vi "Set Object Bounds.vi"(5 "Resize Only? [F]":bool, 7 "Position Only? [F]":bool, 8 "error in (no error)":errorcluster, 9 "rect":T1, 11 "GObject":refnum<vi>) -> (0 "error out":errorcluster, 3 "DUP GObject":refnum<vi>)   [LabVIEW 2013, in "IObject.lvclass"]
uses:
  IObject.lvclass
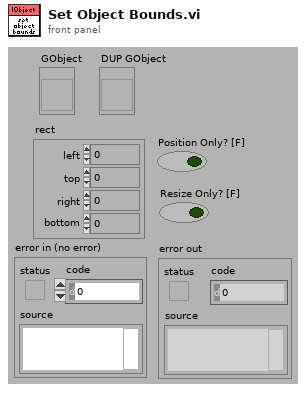
[diagram p1: front panel]
types:
  T1 = cluster{"left":dbl, "top":dbl, "right":dbl, "bottom":dbl}
  T2 = cluster{"left":bool, "top":bool, "right":bool, "bottom":bool}
  T3 = cluster{"left":i32, "top":i32, "right":i32, "bottom":i32}
  T4 = typedef "LVPositionTypeDef.ctl" = cluster{"Left":i32, "Top":i32}
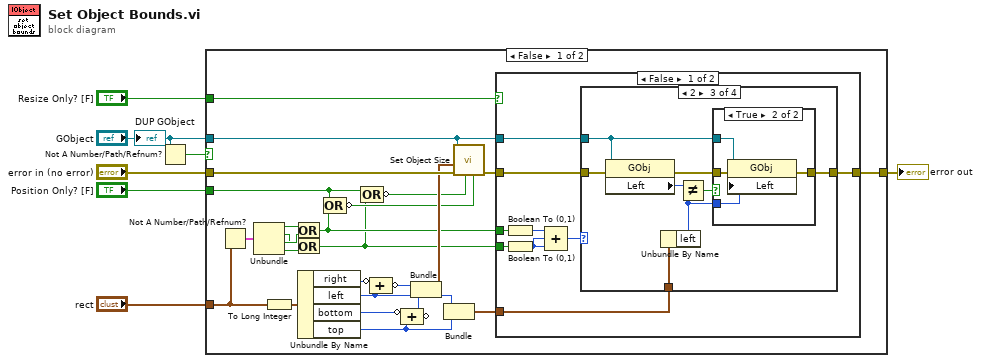
[diagram p0: block diagram]
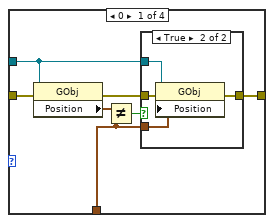
[diagram p2: hidden frame]
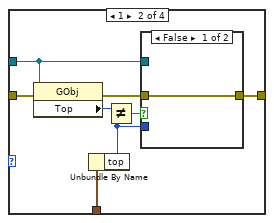
[diagram p4: hidden frame]
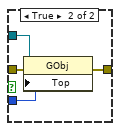
[diagram p5: hidden frame]
diagram:
  n1 = Not A Number/Path/Refnum?(number/path/refnum="GObject") -> (NaN/Path/Refnum?=w1:bool)
  n2 = case shown="False" w1 {
    tunnel: "error in (no error)" -> [w32 w82]
    tunnel: [w31 w82] -> w6
    tunnel: "Position Only? [F]" -> [w10 _]
    tunnel: "Resize Only? [F]" -> [w30 _]
    tunnel: "GObject" -> [w23 _]
    tunnel: "rect" -> [w18 _]
    frame False {
      n3 = Not A Number/Path/Refnum?(number/path/refnum=w18) -> (NaN/Path/Refnum?=w17:T2)
      n4 = Unbundle(w17) -> ("left"=w16:bool, "top"=w14:bool, "right"=w15:bool, "bottom"=w13:bool)
      n5 = To Long Integer(number=w18) -> (32bit integer=w29:T3)
      n6 = Or(x=w16, y=w15) -> (x .or. y?=w9:bool)
      n7 = Or(x=w14, y=w13) -> (x .or. y?=w8:bool)
      n8 = Unbundle By Name(w29) -> ("right"=w28:i32, "left"=w21:i32, "bottom"=w27:i32, "top"=w20:i32)
      n9 = Compound Arithmetic op=OR(w10, w9) -> (invert w12:bool)
      n10 = Compound Arithmetic op=OR(w10, w8) -> (invert w11:bool)
      n11 = Compound Arithmetic op=ADD(invert w28, w21) -> (invert w26:i32)
      n12 = Compound Arithmetic op=ADD(invert w27, w20) -> (invert w25:i32)
      n13 = Bundle(w26, w25) -> (w24:cluster{i32, i32})  [unwired: 1 out]
      n14 = Bundle("left"=w21, "top"=w20) -> (w19:cluster{"left":i32, "top":i32})  [unwired: 1 in]
      n15 = call "Set Object Size.vi"("Set Width?"=w12, "Set Height?"=w11, "error in (no error)"=w32, "Size"=w24, "GObj Refnum"=w23) -> ("error out"=w22:errorcluster)  [unwired: 2 in, 4 out]
      n16 = case shown="False" w30 {
        tunnel: w23 -> [w39 _]
        tunnel: [w40 w81] -> w31
        tunnel: w22 -> [w41 w81]
        tunnel: w19 -> [w38 _]
        tunnel: w9 -> [w37 _]
        tunnel: w8 -> [w36 _]
        frame False {
          n17 = Boolean To (0,1)(Boolean=w37) -> (0, 1=w35:i16)
          n18 = Boolean To (0,1)(Boolean=w36) -> (0, 1=w34:i16)
          n19 = Compound Arithmetic op=ADD(w35, w34, w34) -> (w33:i16)
          n20 = case shown="2" w33 {
            tunnel: w41 -> [w48 w61 w74 w80]
            tunnel: [w45 w58 w71 w80] -> w40
            tunnel: w39 -> [w44 w57 w70 _]
            tunnel: w38 -> [w43 w55 w68 _]
            frame 0 {
              n21 = property class="GObj"(reference=w44, error in=w48) -> (error out=w47:errorcluster, "Position"=w46:T4)  [unwired: 1 out]
              n22 = Not Equal?(x=w46, y=w43) -> (x != y?=w42:bool)
              n23 = case shown="True" w42 {
                tunnel: [w49 w53] -> w45
                tunnel: w44 -> [_ w52]
                tunnel: w47 -> [w49 w51]
                tunnel: w43 -> [_ w50]
                frame False {
                }
                frame True {
                  n24 = property class="GObj"(reference=w52, error in=w51, "Position"=w50) -> (error out=w53:errorcluster)  [unwired: 1 out]
                }
              }
            }
            frame 1 {
              n25 = property class="GObj"(reference=w57, error in=w61) -> (error out=w60:errorcluster, "Top"=w59:i32)  [unwired: 1 out]
              n26 = Unbundle By Name(w55) -> ("top"=w54:i32)
              n27 = Not Equal?(x=w59, y=w54) -> (x != y?=w56:bool)
              n28 = case shown="False" w56 {
                tunnel: [w62 w66] -> w58
                tunnel: w57 -> [_ w65]
                tunnel: w60 -> [w62 w64]
                tunnel: w54 -> [_ w63]
                frame False {
                }
                frame True {
                  n29 = property class="GObj"(reference=w65, error in=w64, "Top"=w63) -> (error out=w66:errorcluster)  [unwired: 1 out]
                }
              }
            }
            frame 2 {
              n30 = property class="GObj"(reference=w70, error in=w74) -> (error out=w73:errorcluster, "Left"=w72:i32)  [unwired: 1 out]
              n31 = Unbundle By Name(w68) -> ("left"=w67:i32)
              n32 = Not Equal?(x=w72, y=w67) -> (x != y?=w69:bool)
              n33 = case shown="True" w69 {
                tunnel: [w75 w79] -> w71
                tunnel: w70 -> [_ w78]
                tunnel: w73 -> [w75 w77]
                tunnel: w67 -> [_ w76]
                frame False {
                }
                frame True {
                  n34 = property class="GObj"(reference=w78, error in=w77, "Left"=w76) -> (error out=w79:errorcluster)  [unwired: 1 out]
                }
              }
            }
            frame 3, Default {
            }
          }
        }
        frame True {
        }
      }
    }
    frame True {
    }
  }
  "error out" <- w6
  "DUP GObject" <- "GObject"
